vi "XIPIN_AXI_IIC_2_0.vi"   [LabVIEW 2017]
doc: "AXI IIC controller\n------------------------------------\n<b>Need License</b> : No\n<b>Interface</b> : AXI4"
uses:
  <vilib>/rvi/XilinxIP/XIPIN_XNode/niFpgaXIPIN.xnode
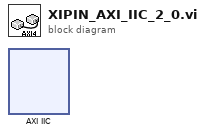
[diagram p0: block diagram]
diagram:
  n1 = xnode ("AXI IIC")() -> ()
